vi "Pega_Tags_cluster_saida.vi"() -> (2 "TipoTag":string[](array[string]), 3 "Array Tags":string[](array[string]))   [LabVIEW 2019]
uses:
  padrao_todos_os_dados_SAIDA.ctl
  padrao_UCM.004.EEL.0300_SAIDA.ctl
  padrao_UCM.004.EEL.0200_SAIDA.ctl
  padrao_INTERNO.ctl
panel:
  in  "todos_os_dados_SAIDA":T1
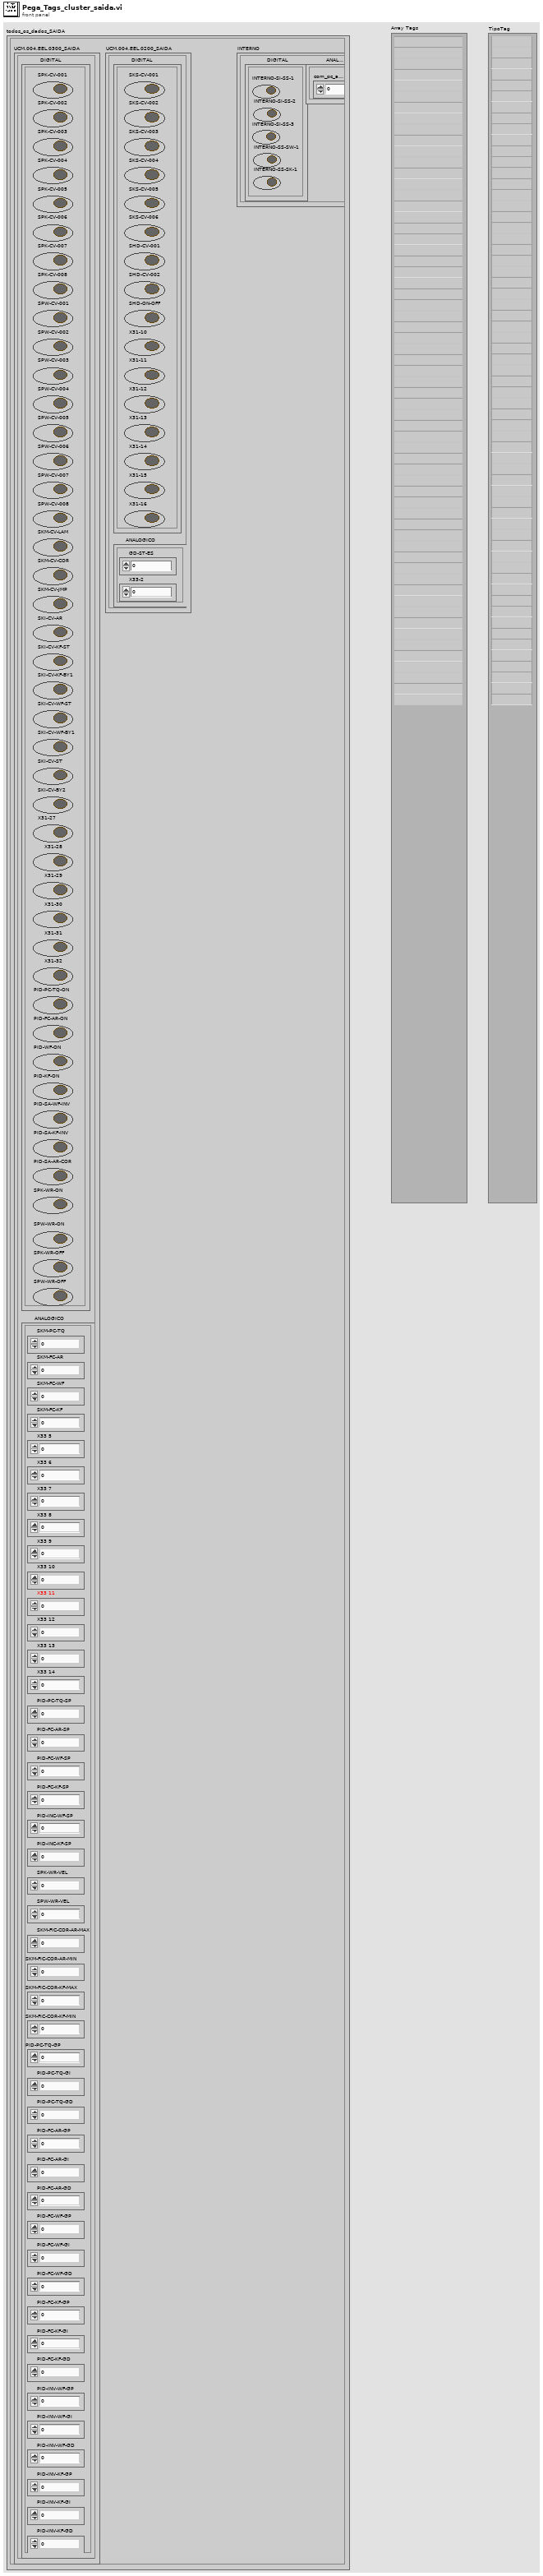
[diagram p1: front panel]
types:
  T1 = typedef "padrao_todos_os_dados_SAIDA.ctl" = cluster{"UCM.004.EEL.0300_SAIDA":T2, "UCM.004.EEL.0200_SAIDA":T3, "INTERNO":T4}
  T2 = typedef "padrao_UCM.004.EEL.0300_SAIDA.ctl" = cluster{"DIGITAL":cluster{"SPK-CV-001":bool, "SPK-CV-002":bool, "SPK-CV-003":bool, "SPK-CV-004":bool, "SPK-CV-005":bool, "SPK-CV-006":bool, "SPK-CV-007":bool, "SPK-CV-008":bool, "SPW-CV-001":bool, "SPW-CV-002":bool, "SPW-CV-003":bool, "SPW-CV-004":bool, "SPW-CV-005":bool, "SPW-CV-006":bool, "SPW-CV-007":bool, "SPW-CV-008":bool, "SKM-CV-LAM":bool, "SKM-CV-COR":bool, "SKM-CV-JMP":bool, "SKI-CV-AR":bool, "SKI-CV-KF-ST":bool, "SKI-CV-KF-BY1":bool, "SKI-CV-WF-ST":bool, "SKI-CV-WF-BY1":bool, "SKI-CV-ST":bool, "SKI-CV-BY2":bool, "X31-27":bool, "X31-28":bool, "X31-29":bool, "X31-30":bool, "X31-31":bool, "X31-32":bool, "PID-PC-TQ-ON":bool, "PID-FC-AR-ON":bool, "PID-WF-ON":bool, "PID-KF-ON":bool, "PID-SA-WF-INV":bool, "PID-SA-KF-INV":bool, "PID-SA-AR-COR":bool, "SPK-WR-ON":bool, "SPW-WR-ON":bool, "SPK-WR-OFF":bool, "SPW-WR-OFF":bool}, "ANALOGICO":cluster{"SKM-PC-TQ":i16, "SKM-FC-AR":i16, "SKM-FC-WF":i16, "SKM-FC-KF":i16, "X33 5":i16, "X33 6":i16, "X33 7":i16, "X33 8":i16, "X33 9":i16, "X33 10":i16, "X33 11":i16, "X33 12":i16, "X33 13":i16, "X33 14":i16, "PID-PC-TQ-SP":i16, "PID-FC-AR-SP":i16, "PID-FC-WF-SP":i16, "PID-FC-KF-SP":i16, "PID-INC-WF-SP":i16, "PID-INC-KF-SP":i16, "SPK-WR-VEL":i32, "SPW-WR-VEL":i32, "SKM-FIC-COR-AR-MAX":dbl, "SKM-FIC-COR-AR-MIN":dbl, "SKM-FIC-COR-KF-MAX":dbl, "SKM-FIC-COR-KF-MIN":dbl, "PID-PC-TQ-GP":dbl, "PID-PC-TQ-GI":dbl, "PID-PC-TQ-GD":dbl, "PID-FC-AR-GP":dbl, "PID-FC-AR-GI":dbl, "PID-FC-AR-GD":dbl, "PID-FC-WF-GP":dbl, "PID-FC-WF-GI":dbl, "PID-FC-WF-GD":dbl, "PID-FC-KF-GP":dbl, "PID-FC-KF-GI":dbl, "PID-FC-KF-GD":dbl, "PID-INV-WF-GP":dbl, "PID-INV-WF-GI":dbl, "PID-INV-WF-GD":dbl, "PID-INV-KF-GP":dbl, "PID-INV-KF-GI":dbl, "PID-INV-KF-GD":dbl}}
  T3 = typedef "padrao_UCM.004.EEL.0200_SAIDA.ctl" = cluster{"DIGITAL":cluster{"SKS-CV-001":bool, "SKS-CV-002":bool, "SKS-CV-003":bool, "SKS-CV-004":bool, "SKS-CV-005":bool, "SKS-CV-006":bool, "SHD-CV-001":bool, "SHD-CV-002":bool, "SHD-ON-OFF":bool, "X31-10":bool, "X31-11":bool, "X31-12":bool, "X31-13":bool, "X31-14":bool, "X31-15":bool, "X31-16":bool}, "ANALOGICO":cluster{"GD-ST-ES":i16, "X33-2":i16}}
  T4 = typedef "padrao_INTERNO.ctl" = cluster{"DIGITAL":cluster{"INTERNO-SI-SS-1":bool, "INTERNO-SI-SS-2":bool, "INTERNO-SI-SS-3":bool, "INTERNO-SS-SW-1":bool, "INTERNO-SS-SK-1":bool}, "ANALOGICO":cluster{"com_pc_analog":dbl}}
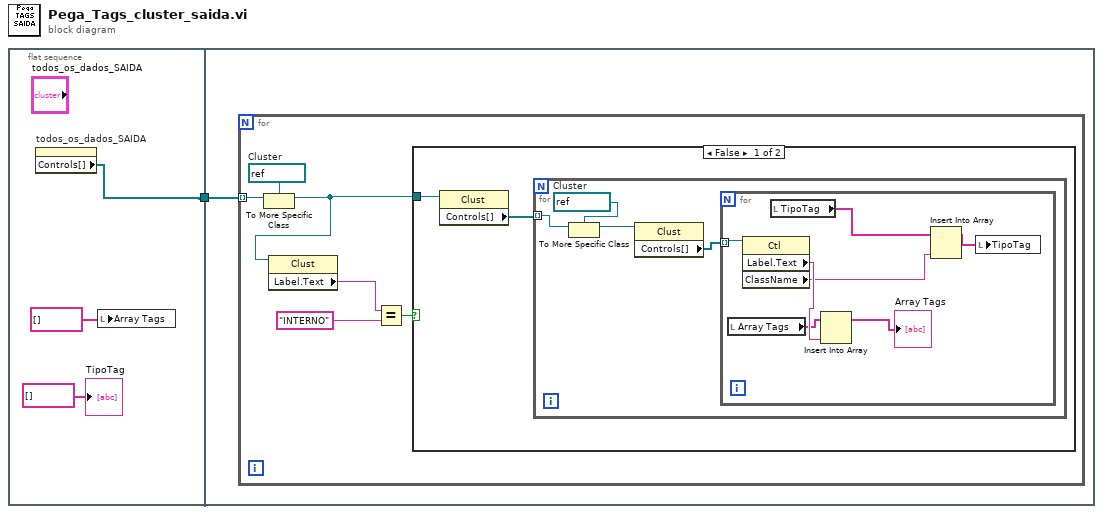
[diagram p0: block diagram]
diagram:
  n1 = flat-sequence {
    tunnel: [w2] -> w1
    tunnel: w1 -> [w5]
    frame #0 {
      n2 = property on="todos_os_dados_SAIDA" class="Clust (strict)"() -> ("Controls[]"=w2:refnum<vi>[])  [unwired: 2 in, 2 out]
      n3 = local write "Array Tags"(string[] [] ("Array")) -> ()
      "TipoTag" <- string[] [] ("Array")
    }
    frame #1 {
      n4 = for {
        tunnel: w5 -> [w10] mode=indexing
        w11 = refnum<vi> refnum  # Cluster
        n5 = To More Specific Class(target class=w11, reference=w10) -> (specific class reference=w6:refnum<vi>)  [unwired: 1 in, 1 out]
        n6 = property on="Property Node" class="Clust"(reference=w6) -> ("Label.Text"=w9:string)  [unwired: 1 in, 2 out]
        n7 = Equal?(x=w9, y="INTERNO") -> (x = y?=w7:bool)
        n8 = case shown="False" w7 {
          tunnel: w6 -> [w13 _]
          frame False {
            n9 = property on="Property Node" class="Clust"(reference=w13) -> ("Controls[]"=w12:refnum<vi>[])  [unwired: 1 in, 2 out]
            n10 = for {
              tunnel: w12 -> [w16] mode=indexing
              w15 = refnum<vi> refnum  # Cluster
              n11 = To More Specific Class(target class=w15, reference=w16) -> (specific class reference=w17:refnum<vi>)  [unwired: 1 in, 1 out]
              n12 = property on="Property Node" class="Clust"(reference=w17) -> ("Controls[]"=w14:refnum<vi>[])  [unwired: 1 in, 2 out]
              n13 = for {
                tunnel: w14 -> [w24] mode=indexing
                n14 = local read "Array Tags"() -> (w21:string[])
                n15 = property class="Ctl"(reference=w24) -> ("Label.Text"=w23:string, "ClassName"=w19:string)  [unwired: 1 in, 2 out]
                n16 = local read "TipoTag"() -> (w20:string[])
                n17 = Insert Into Array(array=w21, new element=w23) -> (→"Array Tags":string[])  [unwired: 1 in]
                n18 = Insert Into Array(array=w20, new element=w19) -> (w18:string[])  [unwired: 1 in]
                n19 = local write "TipoTag"(w18) -> ()
              }
            }
          }
          frame True {
          }
        }
      }
    }
  }
